vi "flat sequence structure.vi"() -> ()   [LabVIEW 2012]
panel:
  out "x/y 2":dbl
  out "x+y 2":dbl
  out "x+y":dbl
  out "x/y":dbl
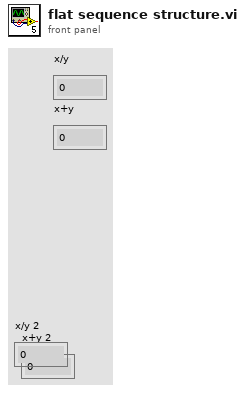
[diagram p1: front panel]
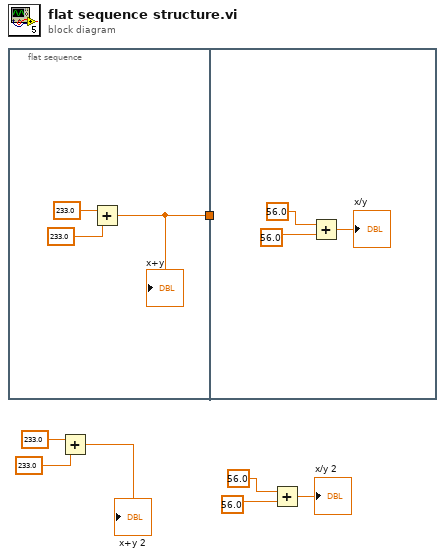
[diagram p0: block diagram]
diagram:
  n1 = flat-sequence {
    tunnel: [w10] -> w7
    tunnel: w7 -> [_]
    frame #0 {
      n2 = Add(x=233.0, y=233.0) -> (x+y=w10:dbl)
      "x+y" <- w10
    }
    frame #1 {
      n3 = Add(x=56.0, y=56.0) -> (x+y=→"x/y":dbl)
    }
  }
  n4 = Add(x=233.0, y=233.0) -> (x+y=→"x+y 2":dbl)
  n5 = Add(x=56.0, y=56.0) -> (x+y=→"x/y 2":dbl)
